vi "Load Project Errors.vi"(8 "error in (no error)":errorcluster, 10 "error file path":path, 11 "project path":path) -> (0 "error out":errorcluster, 2 "canceled?":bool, 3 "error list <top>":variant)   [LabVIEW 2017]
uses:
  Controls/Error Code Window Modes.ctl
  Error List/Scope.ctl
  Error List/Error Code File Properties.ctl
  Error File Management/Error File Management.lvlib
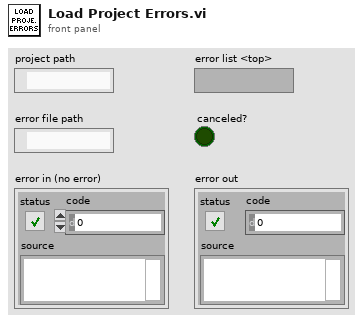
[diagram p1: front panel]
types:
  T1 = typedef "Scope.ctl" = enum16{"project", "global"}
  T2 = typedef "Error Code File Properties.ctl" = cluster{"path":path, "simplified path":string, "name":string, "display name":string, "family name":string, "comment":string, "parsable?":bool, "file modified?":bool}
  T3 = typedef "Error Code Window Modes.ctl" = u8
  T4 = typedef "Error File Management.lvlib/NI Error.ctl" = errorcluster
  T5 = typedef "Error File Management.lvlib/NI Family.ctl" = cluster{"family name":string, "display name":string}
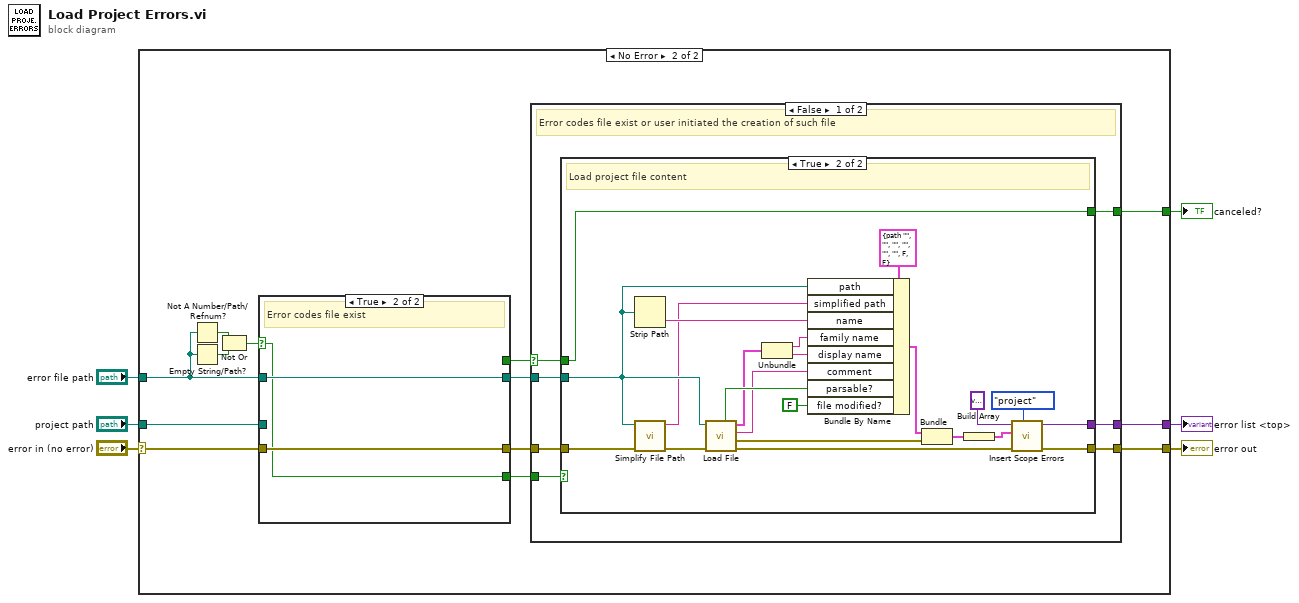
[diagram p0: block diagram]
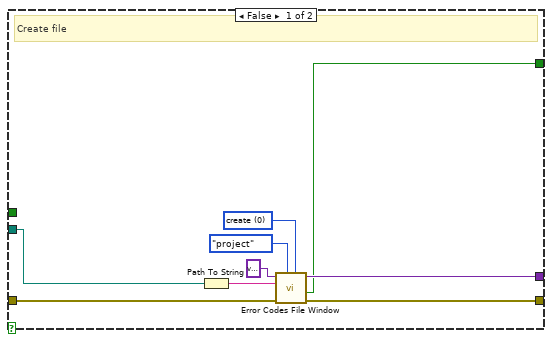
[diagram p3: hidden frame]
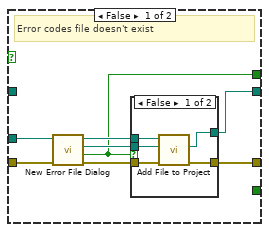
[diagram p5: hidden frame]
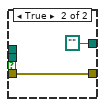
[diagram p6: hidden frame]
diagram:
  n1 = case shown="No Error" "error in (no error)" {
    selector: "error in (no error)" -> [w7 w12]
    tunnel: "project path" -> [_ w16]
    tunnel: "error file path" -> [_ w14]
    tunnel: [w7 w13] -> w3
    tunnel: [_ w8] -> w2
    tunnel: [_ w10] -> w1
    frame Error {
    }
    frame No Error {
      n2 = Not A Number/Path/Refnum?(number/path/refnum=w14) -> (NaN/Path/Refnum?=w19:bool)
      n3 = Empty String/Path?(string/path=w14) -> (empty?=w20:bool)
      n4 = Not Or(1:w20, 2:w19) -> (0:w18:bool)
      n5 = case shown="True" w18 {
        selector: w18 -> [_ w76]
        tunnel: [w64 w78] -> w17
        tunnel: w16 -> [w67 _]
        tunnel: [w68 w77] -> w15
        tunnel: w14 -> [_ w78]
        tunnel: [w62 _] -> w11
        tunnel: w12 -> [w61 w77]
        tunnel: [_ w76] -> w9
        frame False {
          # "Error codes file doesn't exist"
          n6 = call "New Error File Dialog.vi"("error in (no error)"=w61, "project path in"=w67) -> ("error out"=w63:errorcluster, "canceled?"=w62:bool, "file path"=w65:path, "project path dup"=w66:path)  [unwired: 6 in]
          n7 = case shown="False" w62 {
            tunnel: [w73 w75] -> w68
            tunnel: w66 -> [w72 _]
            tunnel: w65 -> [w71 _]
            tunnel: [w70 path ""] -> w64
            tunnel: w63 -> [w69 w75]
            frame False {
              n8 = call "Add File to Project.vi"("error in (no error)"=w69, "file path"=w71, "project path"=w72) -> ("error out"=w73:errorcluster, "file path dup"=w70:path)  [unwired: 6 in, 1 out]
            }
            frame True {
            }
          }
        }
        frame True {
          # "Error codes file exist"
        }
      }
      n9 = case shown="False" w11 {
        selector: w11 -> [w22 w59]
        tunnel: w17 -> [w25 _]
        tunnel: w15 -> [w27 w60]
        tunnel: [w26 w60] -> w13
        tunnel: [w24 _] -> w10
        tunnel: w9 -> [w23 _]
        tunnel: [w21 w59] -> w8
        frame False {
          # "Error codes file exist or user initiated the creation of such file"
          n10 = case shown="True" w23 {
            tunnel: w27 -> [w36 w56]
            tunnel: [w32 w54] -> w26
            tunnel: w25 -> [w30 w46]
            tunnel: [w31 w39] -> w24
            tunnel: w22 -> [_ w37]
            tunnel: [w28 w37] -> w21
            frame False {
              w35 = T3 0 items=["create", "edit"] ("mode")
              # "Create file"
              n11 = Path To String(path=w30) -> (string=w29:string)
              n12 = call "Error Codes File Window.vi"("mode"=w35, "scope"=Scope."project", "error in (no error)"=w36, "owner path"=w29, "error list <top> in"=variant) -> ("error out"=w32:errorcluster, "cancelled?"=w28:bool, "error list <top> out"=w31:variant)  [unwired: 3 in, 1 out]
            }
            frame True {
              # "Load project file content"
              n13 = Strip Path(path=w46) -> (name=w45:string)  [unwired: 1 out]
              n14 = call "Simplify File Path.vi"("error in (no error)"=w56, "full path"=w46) -> ("error out"=w57:errorcluster, "simplified path"=w44:string)  [unwired: 8 in]
              n15 = call "Load File.vi"("error in (no error)"=w57, "error codes file"=w46) -> ("error out"=w55:errorcluster, "errors"=w49:T4[], "comment"=w41:string, "family"=w38:T5, "parsable?"=w58:bool)  [unwired: 5 in]
              n16 = Unbundle(w38) -> ("family name"=w43:string, "display name"=w42:string)
              n17 = Bundle By Name(cluster=T2 {"path"=path "", "simplified path"="", "name"="", "display name"="", "family name"="", "comment"="", "parsable?"=FALSE, "file modified?"=FALSE} ("properties"), "path"=w46, "simplified path"=w44, "name"=w45, "family name"=w43, "display name"=w42, "comment"=w41, "parsable?"=w58, "file modified?"=FALSE) -> (w50:T2)
              n18 = Bundle("properties"=w50, "errors"=w49) -> (w48:cluster{"properties":T2, "errors":T4[]})  [unwired: 1 in]
              n19 = Build Array(w48) -> (w47:cluster{"properties":T2, "errors":T4[]}[])
              n20 = call "Insert Scope Errors.vi"("scope"=Scope."project", "error in (no error)"=w55, "error codes file content"=w47, "error list <top> in"=variant) -> ("error out"=w54:errorcluster, "error list <top> out"=w39:variant)  [unwired: 6 in]
            }
          }
        }
        frame True {
          # "Error codes file doesn't exist and user canceled the creation of such file"
        }
      }
    }
  }
  "error out" <- w3
  "canceled?" <- w2
  "error list <top>" <- w1
